vi "HW handle error.vi"(8 "error in (no error)":T1, 10 "module loopdata":T2, 11 "command":string) -> ()   [LabVIEW 2019, in "HW Control.lvlib"]
uses:
  HW Control.lvlib
  module data.ctl
  SubVIs/mmWave instrument_class/mmWave instrument.lvclass
  SubVIs/Timing_class/Timing.lvclass
  Intertarget communication/UE_slave_class/UE_slave.lvclass
  SubVIs/Shared/Shared.lvlib
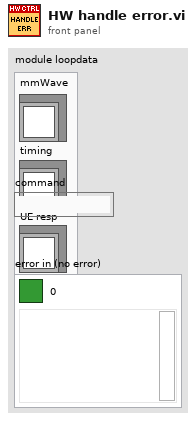
[diagram p1: front panel]
types:
  T1 = cluster{"Boolean Round":bool, "code":i32, "source":string}
  T2 = typedef "HW Control.lvlib/module data.ctl" = cluster{"mmWave":refnum<class "mmWave instrument.lvclass">, "timing":refnum<class "Timing.lvclass">, "UE resp":refnum<class "UE_slave.lvclass">}
  T3 = typedef "mmWave instrument.lvclass/Instrument state.ctl" = enum16{"Off", "Initialization", "Configuration", "Running", "Calibration"}
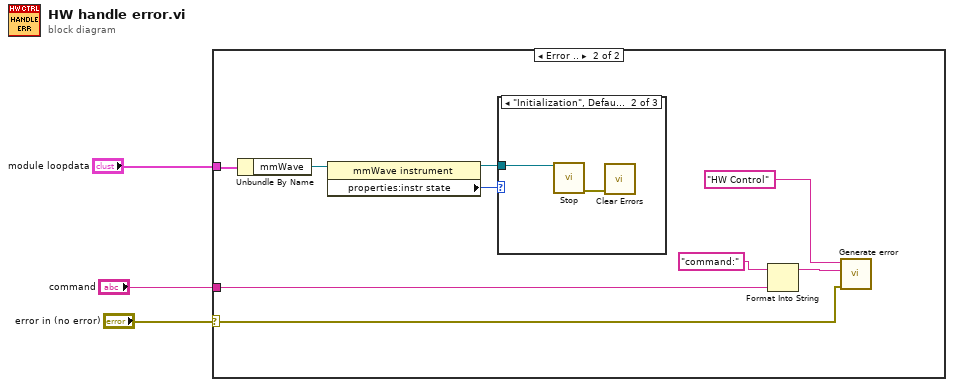
[diagram p0: block diagram]
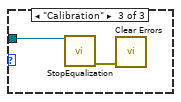
[diagram p4: hidden frame]
diagram:
  n1 = case shown="Error .." "error in (no error)" {
    selector: "error in (no error)" -> [_ w8]
    tunnel: "module loopdata" -> [_ w9]
    tunnel: "command" -> [_ w7]
    frame No Error {
    }
    frame Error {
      n2 = Unbundle By Name(w9) -> ("mmWave"=w6:refnum<class "mmWave instrument.lvclass">)
      n3 = property class="mmWave instrument"(reference=w6) -> (reference out=w4:refnum<class "mmWave instrument.lvclass">, "properties:instr state"=w5:T3)  [unwired: 1 in, 1 out]
      n4 = case shown="\"Initialization\", Default" w5 {
        tunnel: w4 -> [_ w13 w15]
        frame "Off" {
        }
        frame "Initialization", Default {
          n5 = call-dynamic "Stop.vi"("reference in"=w13) -> ("error out"=w14:errorcluster)  [unwired: 9 in, 1 out]
          n6 = call <vilib>:"Clear Errors.vi"("error in (no error)"=w14) -> ()  [unwired: 5 in, 2 out]
        }
        frame "Calibration" {
          n7 = call-dynamic "StopEqualization.vi"("reference in"=w15) -> ("error out"=w16:errorcluster)  [unwired: 9 in, 1 out]
          n8 = call <vilib>:"Clear Errors.vi"("error in (no error)"=w16) -> ()  [unwired: 5 in, 2 out]
        }
      }
      n9 = Format Into String(initial string="command:", w7) -> (resulting string=w11:string)  [unwired: 2 in, 1 out]
      n10 = call "Generate error.vi"("error in (no error)"=w8, "info"=w11, "module"="HW Control") -> ()  [unwired: 8 in, 1 out]
    }
  }
